vi "Get Message Data View VI Ref.vi"(8 "error in (no error)":errorcluster, 11 "Main In":refnum<class "Main.lvclass">) -> (0 "error out":errorcluster, 2 "VI Ref":refnum<vi>, 3 "Main Out":refnum<class "Main.lvclass">)   [LabVIEW 2020, in "Main.lvclass"]
uses:
  Main.lvclass
  Main.lvclass/Main.ctl
  Debug View/Debug View.lvclass
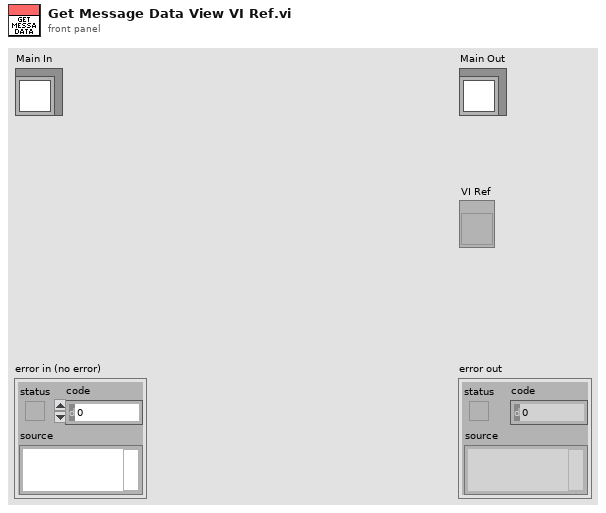
[diagram p1: front panel]
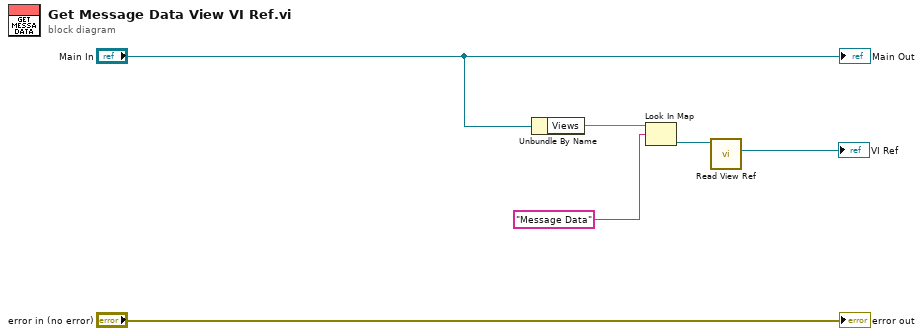
[diagram p0: block diagram]
diagram:
  n1 = Unbundle By Name("Main In") -> ("Views"=w4:map{string, refnum<class "Debug View.lvclass">})
  n2 = Look In Map(map=w4, key="Message Data" ("Name")) -> (value=w2:refnum<class "Debug View.lvclass">)  [unwired: 1 in, 1 out]
  n3 = call "Read View Ref.vi"("Debug View In"=w2) -> ("View Ref"=→"VI Ref":refnum<vi>)  [unwired: 8 in, 2 out]
  "error out" <- "error in (no error)"
  "Main Out" <- "Main In"
